vi "4-1 somma-differenza - vettorelink Ris.vi"(2 "vet b":dbl[](array[numeric])=[1.0, 4.0, 1.0] format="%.2f", 3 "const":dbl=5.0 format="%.2f", 4 "vet a":dbl[](array[numeric])=[1.0, 2.0, 3.0] format="%.2f") -> (0 "vet link":dbl[](array[numeric]) format="%.2f", 1 "vet som-diff":dbl[](array[numeric]) format="%.2f")   [LabVIEW 2012]
doc: "M. Ferrari \n Vector Function Ex"
panel:
  # "1¡ fase\nPER OGNI COMPONENTE DEI VETTORI di INGRESSO \nviene calcolata LA SOMMA se vet a[I] < vet b[I],\naltrimenti LA DIFFERENZA delle due componenti;\nIl risultato sarˆ presente in vet som-diff."
  # "2¡ fase\nL'ultima componente di vet som-diff dovrˆ essere\nsostituita con il valore di const; si vuol creare un nuovo\nvettore, vet link, come risultato della concatenazione\n di vet a, di const(scalare), e di vet som-diff\n(dopo la modifica iniziale sull'ultima componente)."
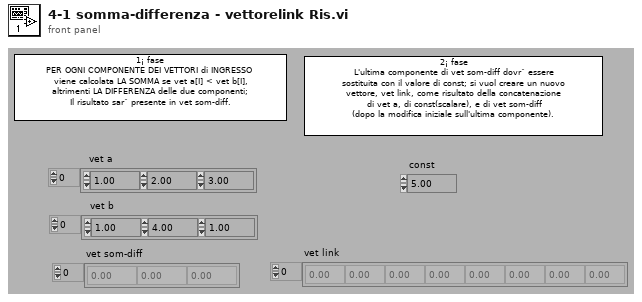
[diagram p1: front panel]
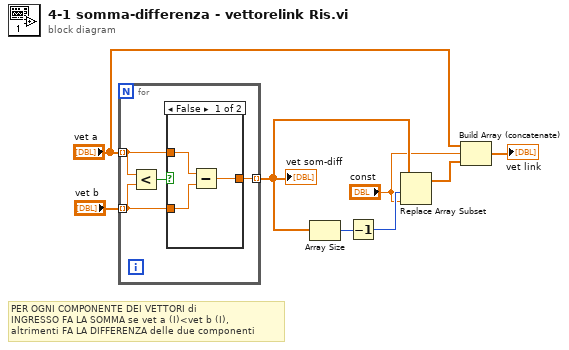
[diagram p0: block diagram]
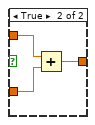
[diagram p2: hidden frame]
diagram:
  # "PER OGNI COMPONENTE DEI VETTORI di\nINGRESSO FA LA SOMMA se vet a (I)<vet b (I),\naltrimenti FA LA DIFFERENZA delle due componenti"
  n1 = for {
    tunnel: "vet a" -> [w11] mode=indexing
    tunnel: "vet b" -> [w10] mode=indexing
    tunnel: [w9] -> w7 mode=indexing
    n2 = Less?(x=w11, y=w10) -> (x < y?=w12:bool)
    n3 = case shown="False" w12 {
      tunnel: w11 -> [w15 w18]
      tunnel: w10 -> [w14 w17]
      tunnel: [w13 w16] -> w9
      frame False {
        n4 = Subtract(x=w15, y=w14) -> (x-y=w13:dbl)
      }
      frame True {
        n5 = Add(x=w18, y=w17) -> (x+y=w16:dbl)
      }
    }
  }
  "vet som-diff" <- w7
  n6 = Array Size(array=w7) -> (size(s)=w6:i32)
  n7 = Decrement(x=w6) -> (x-1=w5:i32)
  n8 = Replace Array Subset(array=w7, new element="const", index=w5) -> (w2:dbl[])
  n9 = Build Array (concatenate)("vet a", "const", w2) -> (→"vet link":dbl[])
